vi "Crosshair placement.vi"(6 "Color":u32(colorbox)=4390744, 9 "y coordinate":sgl, 10 "x coordinate":sgl, 11 "Image":T1) -> (3 "Image Out":T1)   [LabVIEW 2018]
uses:
  <vilib>/vision/Image Controls.llb/IMAQ Image.ctl
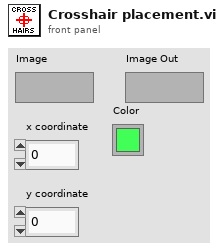
[diagram p1: front panel]
types:
  T1 = typedef "IMAQ Image.ctl" = refnum<image>
  T2 = cluster{"Left":i32, "Top":i32, "Right":i32, "Bottom":i32}
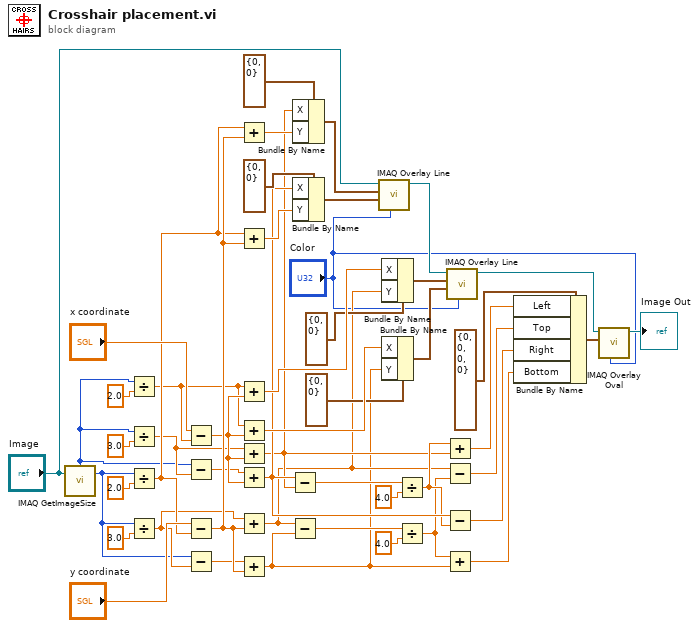
[diagram p0: block diagram]
diagram:
  n1 = call "IMAQ GetImageSize"("Image"="Image") -> ("Y Resolution"=w33:i32, "X Resolution"=w35:i32)  [unwired: 3 in, 1 out]
  n2 = Divide(x=w35, y=2.0) -> (x/y=w38:dbl)
  n3 = Divide(x=w35, y=3.0) -> (x/y=w37:dbl)
  n4 = Divide(x=w33, y=2.0) -> (x/y=w43:dbl)
  n5 = Divide(x=w33, y=3.0) -> (x/y=w34:dbl)
  n6 = Subtract(x="x coordinate", y=w38) -> (x-y=w42:dbl)
  n7 = Subtract(x=w35, y=w37) -> (x-y=w39:dbl)
  n8 = Subtract(x="y coordinate", y=w43) -> (x-y=w46:dbl)
  n9 = Subtract(x=w33, y=w34) -> (x-y=w36:dbl)
  n10 = Add(x=w43, y=w46) -> (x+y=w44:dbl)
  n11 = Add(x=w43, y=w46) -> (x+y=w45:dbl)
  n12 = Add(x=w38, y=w42) -> (x+y=w40:dbl)
  n13 = Add(x=w38, y=w42) -> (x+y=w41:dbl)
  n14 = Add(x=w37, y=w42) -> (x+y=w11:dbl)
  n15 = Add(x=w39, y=w42) -> (x+y=w13:dbl)
  n16 = Add(x=w34, y=w46) -> (x+y=w5:dbl)
  n17 = Add(x=w36, y=w46) -> (x+y=w4:dbl)
  n18 = Subtract(x=w13, y=w11) -> (x-y=w14:dbl)
  n19 = Subtract(x=w5, y=w4) -> (x-y=w7:dbl)
  n20 = Bundle By Name(cluster=cluster{"X":i32, "Y":i32} {"X"=0, "Y"=0} ("Start Point"), "X"=w11, "Y"=w44) -> (w32:cluster{"X":i32, "Y":i32})
  n21 = Bundle By Name(cluster=cluster{"X":i32, "Y":i32} {"X"=0, "Y"=0} ("Start Point"), "X"=w13, "Y"=w45) -> (w31:cluster{"X":i32, "Y":i32})
  n22 = call "IMAQ Overlay Line"("Color"="Color", "End Point"=w31, "Start Point"=w32, "Image"="Image") -> ("Image Out"=w20:T1)  [unwired: 6 in, 1 out]
  n23 = Bundle By Name(cluster=cluster{"X":i32, "Y":i32} {"X"=0, "Y"=0} ("Start Point"), "X"=w40, "Y"=w5) -> (w25:cluster{"X":i32, "Y":i32})
  n24 = Bundle By Name(cluster=cluster{"X":i32, "Y":i32} {"X"=0, "Y"=0} ("Start Point"), "X"=w41, "Y"=w4) -> (w28:cluster{"X":i32, "Y":i32})
  n25 = Divide(x=w14, y=4.0) -> (x/y=w12:dbl)
  n26 = Divide(x=w7, y=4.0) -> (x/y=w8:dbl)
  n27 = Add(x=w12, y=w11) -> (x+y=w9:dbl)
  n28 = Subtract(x=w5, y=w8) -> (x-y=w3:dbl)
  n29 = Subtract(x=w13, y=w12) -> (x-y=w10:dbl)
  n30 = Add(x=w8, y=w4) -> (x+y=w2:dbl)
  n31 = call "IMAQ Overlay Line"("Color"="Color", "End Point"=w28, "Start Point"=w25, "Image"=w20) -> ("Image Out"=w19:T1)  [unwired: 6 in, 1 out]
  n32 = Bundle By Name(cluster=T2 {"Left"=0, "Top"=0, "Right"=0, "Bottom"=0} ("Bounding Rectangle"), "Left"=w9, "Top"=w3, "Right"=w10, "Bottom"=w2) -> (w16:T2)
  n33 = call "IMAQ Overlay Oval"("Color"="Color", "Bounding Rectangle"=w16, "Image"=w19) -> ("Image Out"=→"Image Out":T1)  [unwired: 7 in, 1 out]
